vi "CalculateAM_factor.vi"(5 "b_am":fxp<+/-,16,2>, 7 "a_am":fxp<+/-,16,2>, 11 "AM phase":fxp<+,64,64>) -> (2 "dummy":fxp<+/-,16,0>, 3 "AM_factor":fxp<+/-,16,2>)   [LabVIEW 2013]
doc: "Calculates various combinations on I_in, Q_in and cos(fi) and sin(fi) to be used later to delay the output signal"
uses:
  <vilib>/rvi/FXPMathLib/FxpInterpret/XNode/nifxpmath_Interpret.xnode
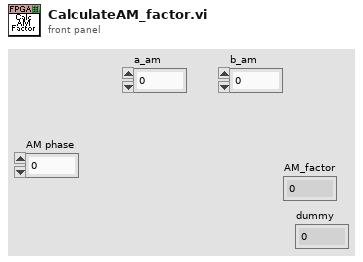
[diagram p1: front panel]
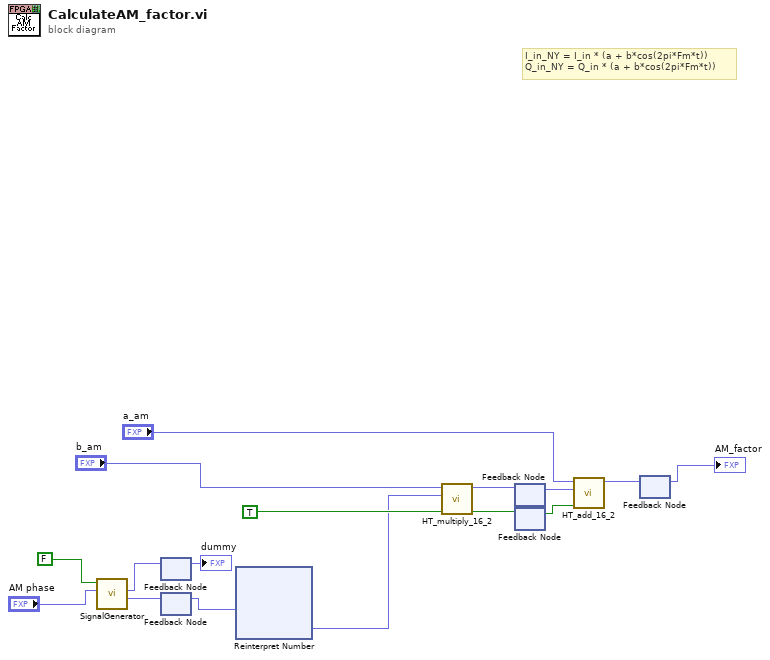
[diagram p0: block diagram]
diagram:
  # "I_in_NY = I_in * (a + b*cos(2pi*Fm*t))\nQ_in_NY = Q_in * (a + b*cos(2pi*Fm*t))"
  n1 = call "SignalGenerator.vi"("phase"="AM phase", "Reset"=FALSE) -> ("Cos"=w7:fxp<+/-,16,0>, "Sin"=w4:fxp<+/-,16,0>)  [unwired: 7 in, 1 out]
  n2 = feedback #1() -> (→"dummy":fxp<+/-,16,0>)  [unwired: 1 in]
  n3 = feedback-in #1(w4) -> ()
  n4 = feedback #2() -> (w2:fxp<+/-,16,0>)  [unwired: 1 in]
  n5 = feedback-in #2(w7) -> ()
  n6 = xnode "Reinterpret Number"("x"=w2) -> ("y"=w1:fxp<+/-,16,2>)
  n7 = call "HT_multiply_16_2.vi"("input valid"=TRUE, "y"=w1, "x"="b_am") -> ("output valid"=w13:bool, "x*y"=w14:fxp<+/-,16,2>)  [unwired: 7 in]
  n8 = feedback #3() -> (w12:fxp<+/-,16,2>)  [unwired: 1 in]
  n9 = feedback-in #3(w14) -> ()
  n10 = feedback #4() -> (w11:bool)  [unwired: 1 in]
  n11 = feedback-in #4(w13) -> ()
  n12 = call "HT_add_16_2.vi"("input valid"=w11, "y"=w12, "x"="a_am") -> ("x+y"=w10:fxp<+/-,16,2>)  [unwired: 7 in, 1 out]
  n13 = feedback #5() -> (→"AM_factor":fxp<+/-,16,2>)  [unwired: 1 in]
  n14 = feedback-in #5(w10) -> ()
